vi "RobotGoToCoord.vi"(1 "X/Y/a Target":T1, 2 "Drive Refnum":string, 3 "X/Y/a Current":T1) -> (0 "Done?":bool)   [LabVIEW 2014]
uses:
  <vilib>/express/express arith-compare/Formula/XNode/ExpressFormulaBlockNode.xnode
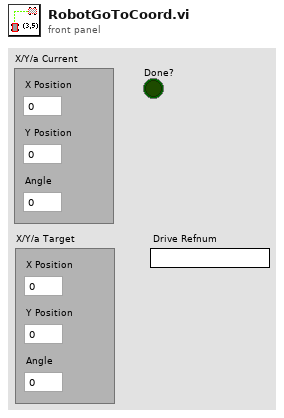
[diagram p1: front panel]
types:
  T1 = cluster{"X Position":dbl, "Y Position":dbl, "Angle":dbl}
  T2 = typedef "WPI_RobotDriveDevRef.ctl" = cluster{"DevStatus":errorcluster, "Motors[]":T3[], "Square Inputs":bool, "Max Output":dbl}
  T3 = typedef "WPI_MotorControlDeviceRef.ctl" = cluster{"DeviceStatus":errorcluster, "Type":T4, "PWM":cluster{"Controller":T5, "PWM Channel":T6, "DeadBand":T7}, "CAN":cluster{"Device Number":u8, "Control Mode":T8, "Semaphore":T9, "Max Vout":dbl, "TalonSRX Control Mode":T10}, "Invert":bool, "TransformRef":T11, "InvTransformRef":T11}
  T4 = typedef "WPI_MotorControlType.ctl" = enum16{"PWM", "CAN", "CANTalonSRX"}
  T5 = typedef "FPGA_TypedefDigitalModule.ctl" = enum16{"Controller 1"}
  T6 = typedef "FPGA_DIOPWMChannel.ctl" = enum8{"PWM 0", "PWM 1", "PWM 2", "PWM 3", "PWM 4", "PWM 5", "PWM 6", "PWM 7", "PWM 8", "PWM 9", "PWM MXP 0", "PWM MXP 1", "PWM MXP 2", "PWM MXP 3", "PWM MXP 4", "PWM MXP 5", "PWM MXP 6", "PWM MXP 7", "PWM MXP 8", "PWM MXP 9", "Invalid"}
  T7 = typedef "WPI_PWMDeadband.ctl" = cluster{"Name":string, "maxPositivePwm":i32, "minPositivePwm":i32, "centerPwm":i32, "maxNegativePwm":i32, "minNegativePwm":i32, "angularRange":u16}
  T8 = typedef "WPI_CANJaguar_ControlMode.ctl" = enum8{"Percent VBus", "Current", "Speed", "Position", "Voltage"}
  T9 = typedef "Semaphore RefNum" = refnum<k1>
  T10 = typedef "WPI_CANTalonSRX_APIControlMode.ctl" = enum8{"Percent VBus", "Speed", "Position", "Slave", "Unchanged / Invalid"}
  T11 = typedef "WPI_PWMTransform_ConPane.ctl" = refnum<vi>
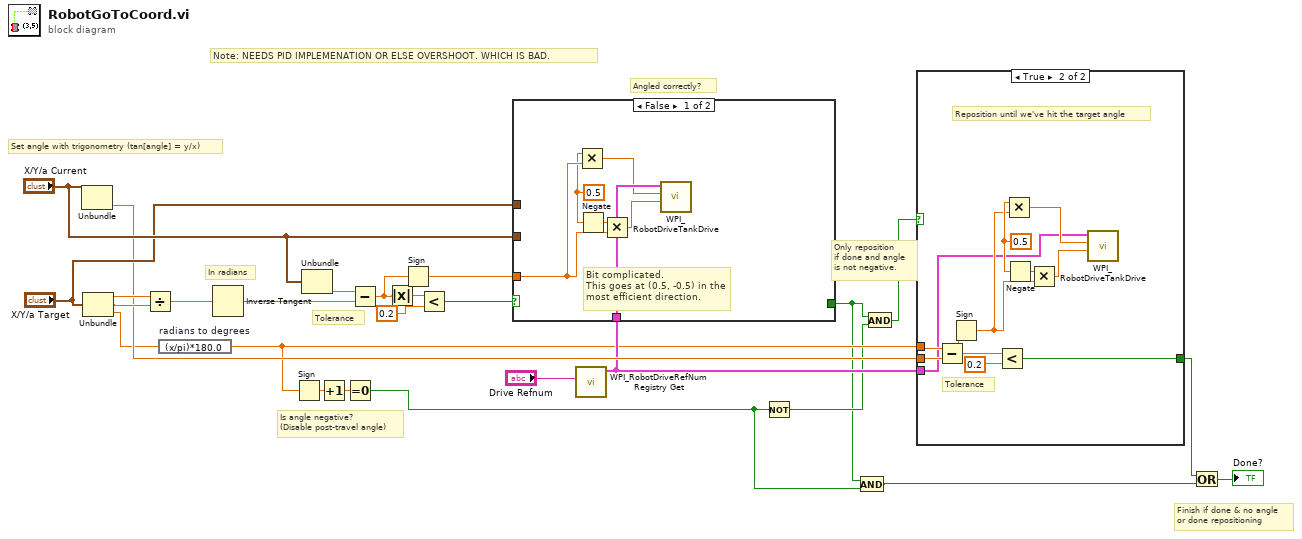
[diagram p0: block diagram]
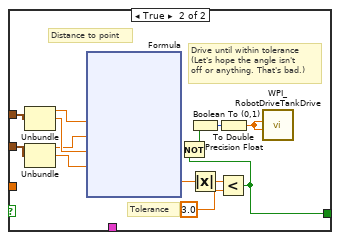
[diagram p3: hidden frame]
diagram:
  # "Finish if done & no angle\nor done repositioning"
  # "Only reposition\nif done and angle\nis not negative."
  # "Is angle negative?\n(Disable post-travel angle)"
  # "Tolerance"
  # "Angled correctly?"
  # "Note: NEEDS PID IMPLEMENATION OR ELSE OVERSHOOT. WHICH IS BAD."
  # "In radians"
  # "Set angle with trigonometry (tan[angle] = y/x)"
  n1 = Unbundle("X/Y/a Current") -> ("Angle"=w13:dbl)  [unwired: 2 out]
  n2 = Unbundle("X/Y/a Target") -> ("X Position"=w25:dbl, "Y Position"=w21:dbl, "Angle"=w11:dbl)
  n3 = Divide(x=w25, y=w21) -> (x/y=w26:dbl)
  n4 = expression code="(x/pi)*180.0" "radians to degrees"(w11) -> (w6:dbl)
  n5 = Inverse Tangent(1:w26) -> (0:w23:dbl)
  n6 = Sign(1:w6) -> (0:w8:dbl)
  n7 = Unbundle("X/Y/a Current") -> ("Angle"=w20:dbl)  [unwired: 2 out]
  n8 = Increment(x=w8) -> (x+1=w7:dbl)
  n9 = Equal To 0?(x=w7) -> (x = 0?=w2:bool)
  n10 = Subtract(x=w20, y=w23) -> (x-y=w16:dbl)
  n11 = Absolute Value(x=w16) -> (abs(x)=w15:dbl)
  n12 = Sign(1:w16) -> (0:w17:dbl)
  n13 = Less?(x=w15, y=0.2) -> (x < y?=w19:bool)
  n14 = call <vilib>:"WPI_RobotDriveRefNum Registry Get.vi"("refnum name"="Drive Refnum") -> ("RobotDriveDevRef"=w12:T2)  [unwired: 9 in, 1 out]
  n15 = case shown="False" w19 {
    tunnel: w12 -> [w29 _]
    tunnel: w17 -> [w32 _]
    tunnel: [_ w36] -> w1
    tunnel: "X/Y/a Target" -> [_ w43]
    tunnel: "X/Y/a Current" -> [_ w40]
    frame False {
      w31 = 0.5
      # "Bit complicated.\nThis goes at (0.5, -0.5) in the most efficient direction."
      n16 = Multiply(x=w31, y=w32) -> (x*y=w28:dbl)
      n17 = Negate(x=w31) -> (-x=w30:dbl)
      n18 = Multiply(x=w30, y=w32) -> (x*y=w27:dbl)
      n19 = call <vilib>:"WPI_RobotDriveTankDrive.vi"("Right axis value"=w27, "Left axis value"=w28, "RobotDriveDevRef"=w29) -> ()  [unwired: 6 in, 3 out]
    }
    frame True {
      # "Drive until within tolerance\n(Let's hope the angle isn't\noff or anything. That's bad.)"
      # "Tolerance"
      # "Distance to point"
      n20 = Unbundle(w43) -> ("X Position"=w42:dbl, "Y Position"=w41:dbl)  [unwired: 1 out]
      n21 = Unbundle(w40) -> ("X Position"=w39:dbl, "Y Position"=w38:dbl)  [unwired: 1 out]
      n22 = xnode "Formula"("X1"=w42, "X2"=w39, "Y1"=w41, "Y2"=w38) -> ("Result"=w37:dbl)  [unwired: 1 in, 1 out]
      n23 = Absolute Value(x=w37) -> (abs(x)=w44:dbl)
      n24 = Less?(x=w44, y=3.0) -> (x < y?=w36:bool)
      n25 = Not(x=w36) -> (.not. x?=w35:bool)
      n26 = Boolean To (0,1)(Boolean=w35) -> (0, 1=w34:i16)
      n27 = To Double Precision Float(number=w34) -> (double precision float=w33:dbl)
      n28 = call <vilib>:"WPI_RobotDriveTankDrive.vi"("Right axis value"=w33, "Left axis value"=w33) -> ()  [unwired: 7 in, 3 out]
    }
  }
  n29 = Not(x=w2) -> (.not. x?=w5:bool)
  n30 = And(x=w1, y=w2) -> (x .and. y?=w3:bool)
  n31 = And(x=w1, y=w5) -> (x .and. y?=w4:bool)
  n32 = case shown="True" w4 {
    tunnel: w6 -> [_ w68]
    tunnel: w13 -> [_ w67]
    tunnel: w12 -> [_ w61]
    tunnel: [_ w60] -> w9
    frame False {
      # "There is no falsehood.\nThere is only the truth."
    }
    frame True {
      w66 = 0.5
      # "Reposition until we've hit the target angle"
      # "Tolerance"
      n33 = Subtract(x=w68, y=w67) -> (x-y=w70:dbl)
      n34 = Sign(1:w70) -> (0:w62:dbl)
      n35 = Less?(x=w70, y=0.2) -> (x < y?=w60:bool)
      n36 = Multiply(x=w66, y=w62) -> (x*y=w64:dbl)
      n37 = Negate(x=w66) -> (-x=w65:dbl)
      n38 = Multiply(x=w65, y=w62) -> (x*y=w63:dbl)
      n39 = call <vilib>:"WPI_RobotDriveTankDrive.vi"("Right axis value"=w63, "Left axis value"=w64, "RobotDriveDevRef"=w61) -> ()  [unwired: 6 in, 3 out]
    }
  }
  n40 = Or(x=w9, y=w3) -> (x .or. y?=→"Done?":bool)
